vi "exercise 3-6.vi"() -> ()   [LabVIEW 2014]
panel:
  out "Output Temperature":dbl
  in  "Input Temperature":dbl
  in  "Enum":enum16{"C to F", "F to C", "C to K", "F to K"}(ring)
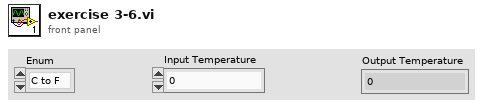
[diagram p1: front panel]
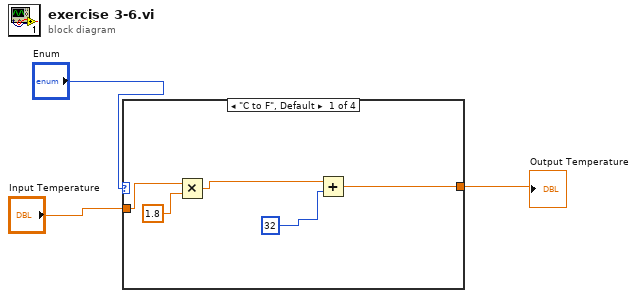
[diagram p0: block diagram]
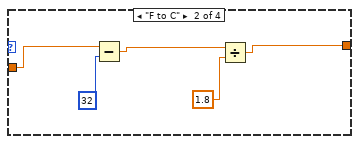
[diagram p2: hidden frame]
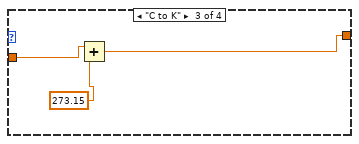
[diagram p3: hidden frame]
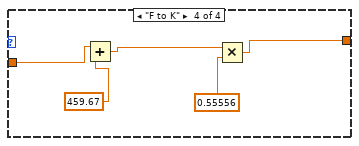
[diagram p4: hidden frame]
diagram:
  n1 = case shown="\"C to F\", Default" "Enum" {
    tunnel: "Input Temperature" -> [w8 w13 w16 w21]
    tunnel: [w4 w9 w14 w17] -> w1
    frame "C to F", Default {
      n2 = Multiply(x=w8, y=1.8) -> (x*y=w6:dbl)
      n3 = Add(x=w6, y=32) -> (x+y=w4:dbl)
    }
    frame "F to C" {
      n4 = Subtract(x=w13, y=32) -> (x-y=w11:dbl)
      n5 = Divide(x=w11, y=1.8) -> (x/y=w9:dbl)
    }
    frame "C to K" {
      n6 = Add(x=w16, y=273.15) -> (x+y=w14:dbl)
    }
    frame "F to K" {
      n7 = Add(x=w21, y=459.67) -> (x+y=w19:dbl)
      n8 = Multiply(x=w19, y=0.55556) -> (x*y=w17:dbl)
    }
  }
  "Output Temperature" <- w1
